vi "Day 07 (Part Two).vi"() -> ()   [LabVIEW 2021]
uses:
  4279ecf5-67f9-43a7-b6b3-78b14aefd003.vi
  4046d748-ad09-4f5d-82b9-a1e726cceff7.vi
  <userlib>/_OpenG.lib/array/array.llb/Sort 2D Array (I32)__ogtk.vi
  <vilib>/Comparison/Less/Less Functor/Less Functor.lvclass
panel:
  out "result":i32
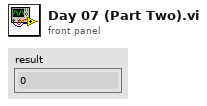
[diagram p1: front panel]
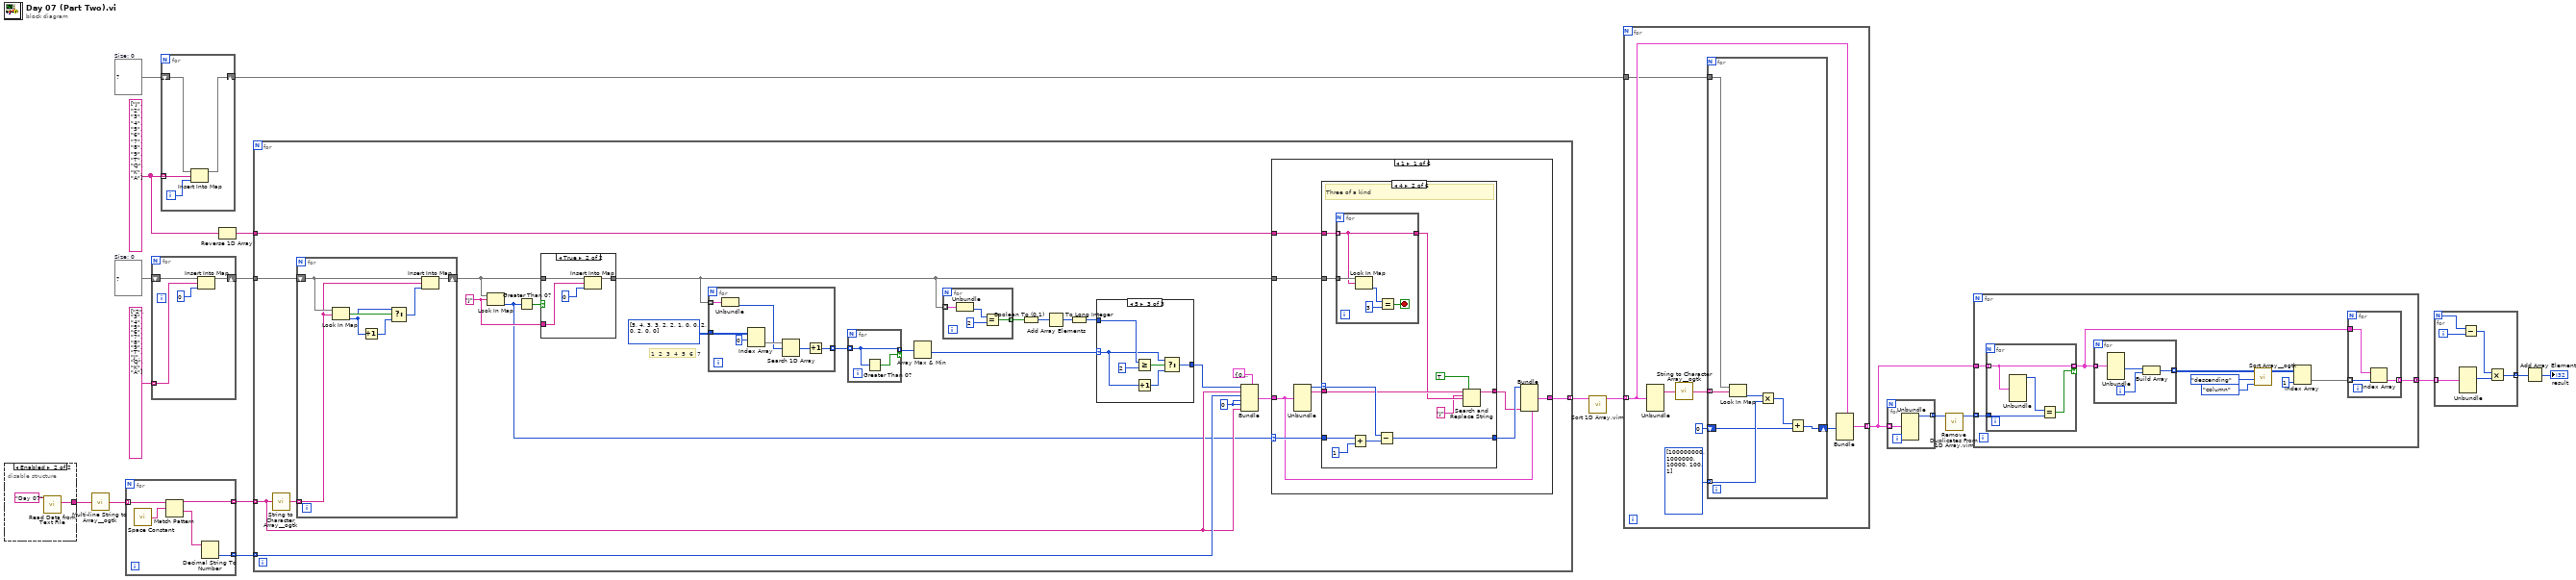
[diagram p0: block diagram]
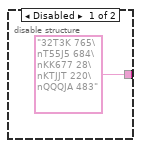
[diagram p2: hidden frame]
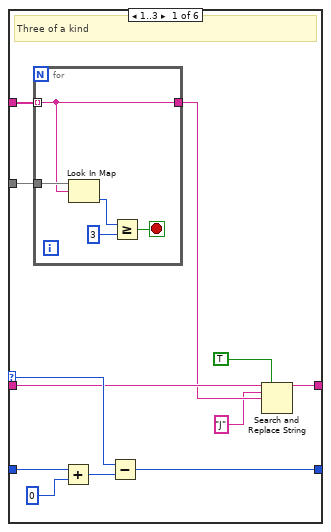
[diagram p3: hidden frame]
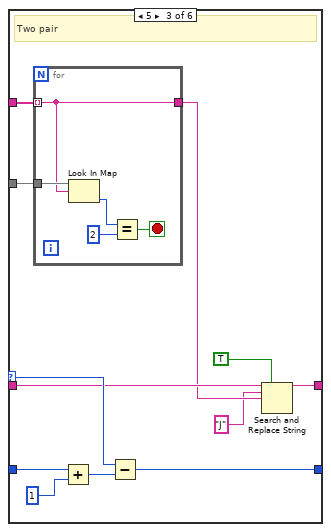
[diagram p4: hidden frame]
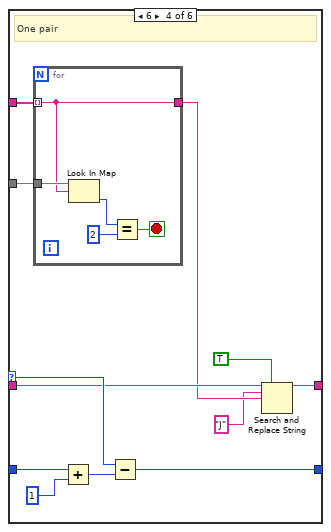
[diagram p5: hidden frame]
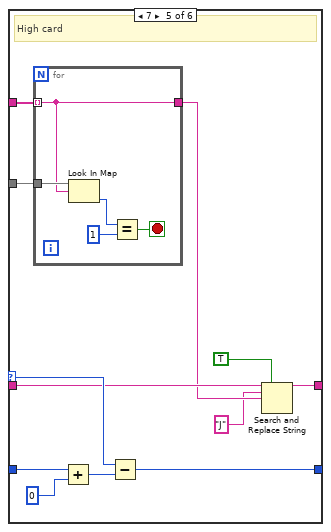
[diagram p6: hidden frame]
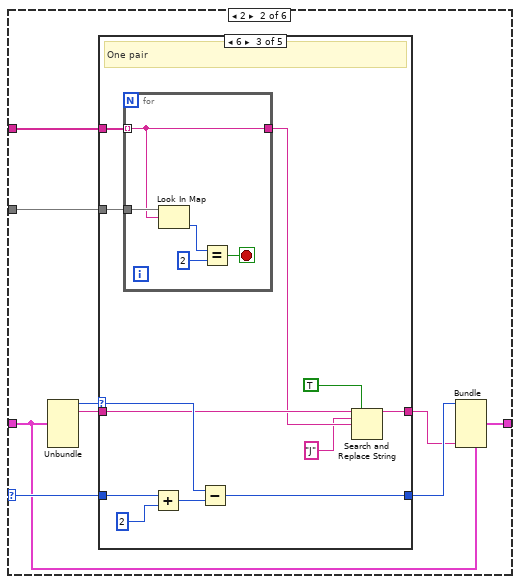
[diagram p8: hidden frame]
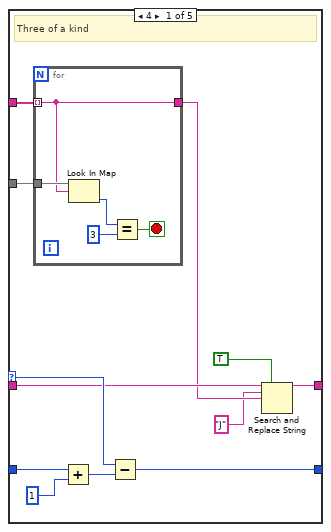
[diagram p9: hidden frame]
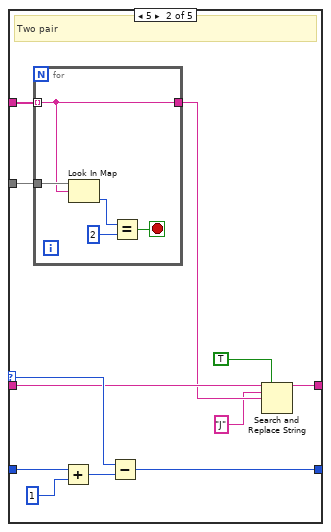
[diagram p10: hidden frame]
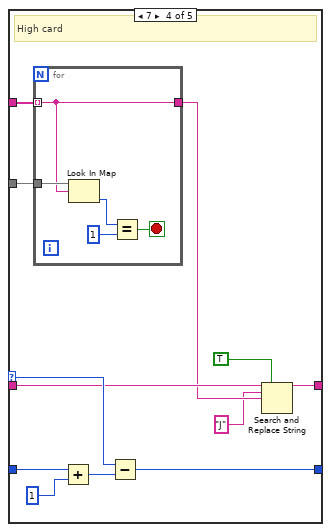
[diagram p11: hidden frame]
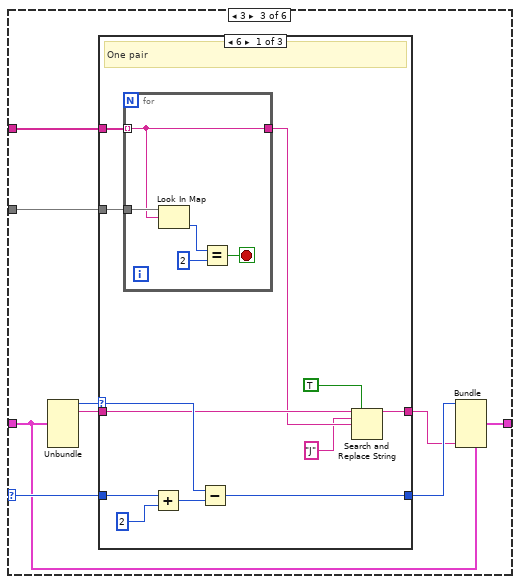
[diagram p13: hidden frame]
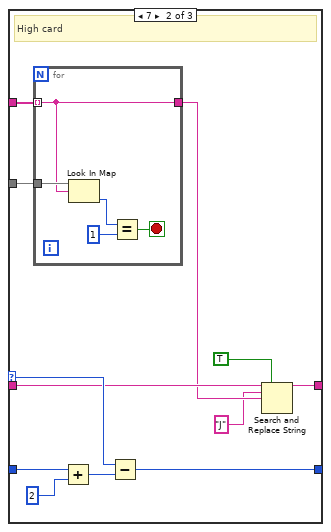
[diagram p14: hidden frame]
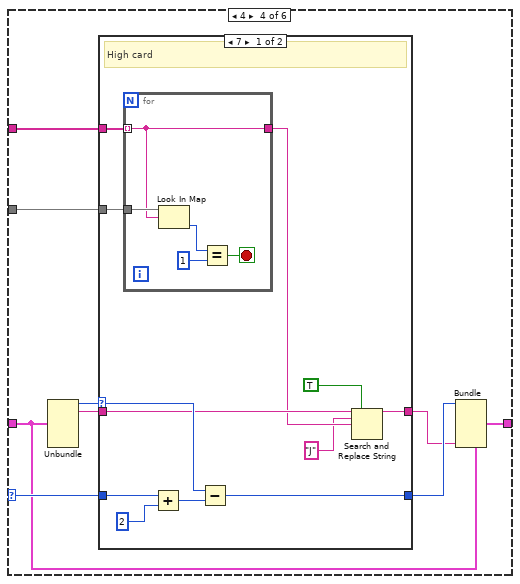
[diagram p16: hidden frame]
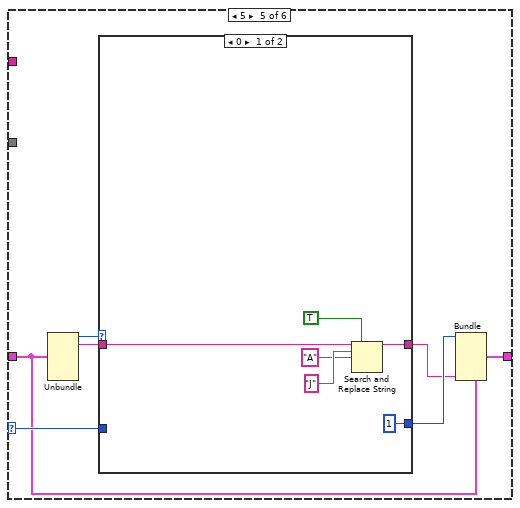
[diagram p18: hidden frame]
diagram:
  w2 = string[] ["J", "2", "3", "4", "5", "6", "7", "8", "9", "T", "Q", "K", "A"]
  w4 = map{string, i32} {}  # Size: 0
  w16 = map{string, i32} {}  # Size: 0
  n1 = disable-structure shown="Enabled" {
    disable-tunnel: ["32T3K 765\nT55J5 684\nKK677 28\nKTJJT 220\nQQQJA 483" w22] -> w19
    frame Disabled {
    }
    frame Enabled {
      n2 = call "Read Data from Text File.vi"("Subfolder"="Day 07") -> ("data"=w22:string)  [unwired: 10 in]
    }
  }
  n3 = call <userlib>:"Multi-line String to Array__ogtk.vi"("string"=w19) -> ("lines"=w18:string[])
  n4 = for {
    tunnel: w18 -> [w27] mode=indexing
    tunnel: [w25] -> w17 mode=indexing
    tunnel: [w23] -> w14 mode=indexing
    n5 = call <vilib>:"Space Constant.vi"() -> ("String"=w26:string)
    n6 = Match Pattern(string=w27, regular expression=w26) -> (before substring=w25:string, after substring=w24:string)  [unwired: 1 in, 2 out]
    n7 = Decimal String To Number(string=w24) -> (number=w23:i32)  [unwired: 2 in, 1 out]
  }
  n8 = for {
    shift-right: [w30] -> w5
    shift-left: w16 -> [w31]
    tunnel: string[] ["2", "3", "4", "5", "6", "7", "8", "9", "T", "J", "Q", "K", "A"] -> [w28] mode=indexing
    n9 = Insert Into Map(map in=w31, key=w28, value=0) -> (map out=w30:map{string, i32})  [unwired: 2 out]
  }
  n10 = for {
    shift-right: [w33] -> w3
    shift-left: w4 -> [w34]
    tunnel: w2 -> [w35] mode=indexing
    i -> [w32]
    n11 = Insert Into Map(map in=w34, key=w35, value=w32) -> (map out=w33:map{string, i32})  [unwired: 2 out]
  }
  n12 = Reverse 1D Array(array=w2) -> (reversed array=w1:string[])
  n13 = for {
    tunnel: w17 -> [w41] mode=indexing
    tunnel: w5 -> [w57]
    tunnel: [w38] -> w15 mode=indexing
    tunnel: w14 -> [w52] mode=indexing
    tunnel: w1 -> [w36]
    w45 = "J" ("key")
    w47 = 0
    # "1  2  3  4  5  6  7"
    n14 = call <userlib>:"String to Character Array__ogtk.vi"("Input String"=w41) -> ("Character Array"=w58:string[])
    n15 = for {
      tunnel: w58 -> [w315] mode=indexing
      shift-right: [w313] -> w44
      shift-left: w57 -> [w316]
      n16 = Look In Map(map=w316, key=w315) -> (key not found?=w319:bool, value=w317:i32)  [unwired: 1 in]
      n17 = Increment(x=w317) -> (x+1=w318:i32)
      n18 = Select(t=w317, s=w319, f=w318) -> (s? t:f=w314:i32)
      n19 = Insert Into Map(map in=w316, key=w315, value=w314) -> (map out=w313:map{string, i32})  [unwired: 2 out]
    }
    n20 = Look In Map(map=w44, key=w45) -> (value=w40:i32)  [unwired: 1 in, 1 out]
    n21 = Greater Than 0?(x=w40) -> (x > 0?=w46:bool)
    n22 = case shown="True" w46 {
      tunnel: w44 -> [w320 w324]
      tunnel: [w320 w323] -> w37
      tunnel: w45 -> [_ w322]
      frame False {
      }
      frame True {
        n23 = Insert Into Map(map in=w324, key=w322, value=0) -> (map out=w323:map{string, i32})  [unwired: 2 out]
      }
    }
    n24 = for {
      tunnel: w37 -> [w331] mode=indexing
      tunnel: i32[][] [[5, 4, 3, 3, 2, 2, 1], [0, 0, 2, 0, 2, 0, 0]] -> [w330]
      tunnel: [w325] -> w56 mode=indexing
      n25 = Unbundle(w331) -> (w327:i32)  [unwired: 1 out]
      n26 = Index Array(array=w330, index (row)=0) -> (element=w328:i32[])  [unwired: 1 in]
      n27 = Search 1D Array(1D array=w328, element=w327) -> (index of element=w326:i32)  [unwired: 1 in]
      n28 = Increment(x=w326) -> (x+1=w325:i32)
    }
    n29 = for {
      tunnel: w56 -> [w333] mode=indexing
      tunnel: [w333] -> w55 mode=indexing if=w332
      n30 = Greater Than 0?(x=w333) -> (x > 0?=w332:bool)
    }
    n31 = Array Max & Min(array=w55) -> (min value=w43:i32)  [unwired: 3 out]
    n32 = for {
      tunnel: w37 -> [w350] mode=indexing
      tunnel: [w347] -> w51 mode=indexing
      n33 = Unbundle(w350) -> (w349:i32)  [unwired: 1 out]
      n34 = Equal?(x=w349, y=2) -> (x = y?=w347:bool)
    }
    n35 = Boolean To (0,1)(Boolean=w51) -> (0, 1=w50:i16[])
    n36 = Add Array Elements(numeric array=w50) -> (sum=w49:i16)
    n37 = To Long Integer(number=w49) -> (32bit integer=w48:i32)
    n38 = case shown="5" w43 {
      selector: w43 -> [w334 w336 w342]
      tunnel: w48 -> [_ w339 w345]
      tunnel: [w334 w335 w341] -> w42
      frame Default {
      }
      frame 3 {
        n39 = Greater Or Equal?(x=w339, y=1) -> (x >= y?=w337:bool)
        n40 = Increment(x=w336) -> (x+1=w338:i32)
        n41 = Select(t=w336, s=w337, f=w338) -> (s? t:f=w335:i32)
      }
      frame 5 {
        n42 = Greater Or Equal?(x=w345, y=2) -> (x >= y?=w343:bool)
        n43 = Increment(x=w342) -> (x+1=w344:i32)
        n44 = Select(t=w342, s=w343, f=w344) -> (s? t:f=w341:i32)
      }
    }
    n45 = Bundle(cluster=cluster{i32, string, i32, i32, i32, string} {0, "", 0, 0, 0, ""}, w42, w41, w52, w47, w47, w41) -> (w39:cluster{i32, string, i32, i32, i32, string})
    n46 = case shown="1" w40 {
      selector: w40 -> [w66 w160 w237 w280 w304 _]
      tunnel: w39 -> [w63 w157 w234 w277 w302 w312]
      tunnel: [w60 w154 w231 w274 w299 w312] -> w38
      tunnel: w37 -> [w65 w159 w236 w279 _ _]
      tunnel: w36 -> [w59 w153 w230 w273 _ _]
      frame 1 {
        n47 = Unbundle(w63) -> (w67:i32, w64:string)  [unwired: 4 out]
        n48 = case shown="4" w67 {
          selector: w67 -> [w78 w95 w112 w129 w146 _]
          tunnel: w66 -> [w71 w88 w105 w122 w139 _]
          tunnel: w65 -> [w79 w96 w113 w130 w147 _]
          tunnel: w64 -> [w77 w94 w111 w128 w145 _]
          tunnel: [w73 w90 w107 w124 w141 _] -> w61
          tunnel: [w72 w89 w106 w123 w140 _] -> w62
          tunnel: w59 -> [w68 w85 w102 w119 w136 _]
          frame 1..3 {
            # "Three of a kind"
            n49 = for {
              tunnel: [w81] -> w76
              tunnel: w79 -> [w83]
              tunnel: w68 -> [w81] mode=indexing
              stop <- w80 stop-if-true
              n50 = Look In Map(map=w83, key=w81) -> (value=w82:i32)  [unwired: 1 in, 1 out]
              n51 = Greater Or Equal?(x=w82, y=3) -> (x >= y?=w80:bool)
            }
            n52 = Add(x=w71, y=0) -> (x+y=w70:i32)
            n53 = Subtract(x=w78, y=w70) -> (x-y=w72:i32)
            n54 = Search and Replace String(replace all?=TRUE ("replace all? (F)"), input string=w77, search string="J", replace string=w76) -> (result string=w73:string)  [unwired: 4 in, 3 out]
          }
          frame 4 {
            # "Three of a kind"
            n55 = for {
              tunnel: [w98] -> w93
              tunnel: w96 -> [w100]
              tunnel: w85 -> [w98] mode=indexing
              stop <- w97 stop-if-true
              n56 = Look In Map(map=w100, key=w98) -> (value=w99:i32)  [unwired: 1 in, 1 out]
              n57 = Equal?(x=w99, y=3) -> (x = y?=w97:bool)
            }
            n58 = Add(x=w88, y=1) -> (x+y=w87:i32)
            n59 = Subtract(x=w95, y=w87) -> (x-y=w89:i32)
            n60 = Search and Replace String(replace all?=TRUE ("replace all? (F)"), input string=w94, search string="J", replace string=w93) -> (result string=w90:string)  [unwired: 4 in, 3 out]
          }
          frame 5 {
            # "Two pair"
            n61 = for {
              tunnel: [w115] -> w110
              tunnel: w113 -> [w117]
              tunnel: w102 -> [w115] mode=indexing
              stop <- w114 stop-if-true
              n62 = Look In Map(map=w117, key=w115) -> (value=w116:i32)  [unwired: 1 in, 1 out]
              n63 = Equal?(x=w116, y=2) -> (x = y?=w114:bool)
            }
            n64 = Add(x=w105, y=1) -> (x+y=w104:i32)
            n65 = Subtract(x=w112, y=w104) -> (x-y=w106:i32)
            n66 = Search and Replace String(replace all?=TRUE ("replace all? (F)"), input string=w111, search string="J", replace string=w110) -> (result string=w107:string)  [unwired: 4 in, 3 out]
          }
          frame 6 {
            # "One pair"
            n67 = for {
              tunnel: [w132] -> w127
              tunnel: w130 -> [w134]
              tunnel: w119 -> [w132] mode=indexing
              stop <- w131 stop-if-true
              n68 = Look In Map(map=w134, key=w132) -> (value=w133:i32)  [unwired: 1 in, 1 out]
              n69 = Equal?(x=w133, y=2) -> (x = y?=w131:bool)
            }
            n70 = Add(x=w122, y=1) -> (x+y=w121:i32)
            n71 = Subtract(x=w129, y=w121) -> (x-y=w123:i32)
            n72 = Search and Replace String(replace all?=TRUE ("replace all? (F)"), input string=w128, search string="J", replace string=w127) -> (result string=w124:string)  [unwired: 4 in, 3 out]
          }
          frame 7 {
            # "High card"
            n73 = for {
              tunnel: [w149] -> w144
              tunnel: w147 -> [w151]
              tunnel: w136 -> [w149] mode=indexing
              stop <- w148 stop-if-true
              n74 = Look In Map(map=w151, key=w149) -> (value=w150:i32)  [unwired: 1 in, 1 out]
              n75 = Equal?(x=w150, y=1) -> (x = y?=w148:bool)
            }
            n76 = Add(x=w139, y=0) -> (x+y=w138:i32)
            n77 = Subtract(x=w146, y=w138) -> (x-y=w140:i32)
            n78 = Search and Replace String(replace all?=TRUE ("replace all? (F)"), input string=w145, search string="J", replace string=w144) -> (result string=w141:string)  [unwired: 4 in, 3 out]
          }
          frame Default {
          }
        }
        n79 = Bundle(cluster=w63, w62, w61) -> (w60:cluster{i32, string, i32, i32, i32, string})  [unwired: 4 in]
      }
      frame 2 {
        n80 = Unbundle(w157) -> (w161:i32, w158:string)  [unwired: 4 out]
        n81 = case shown="6" w161 {
          selector: w161 -> [w172 w189 w206 w223 _]
          tunnel: w160 -> [w165 w182 w199 w216 _]
          tunnel: w159 -> [w173 w190 w207 w224 _]
          tunnel: w158 -> [w171 w188 w205 w222 _]
          tunnel: [w167 w184 w201 w218 _] -> w155
          tunnel: [w166 w183 w200 w217 _] -> w156
          tunnel: w153 -> [w162 w179 w196 w213 _]
          frame 4 {
            # "Three of a kind"
            n82 = for {
              tunnel: [w175] -> w170
              tunnel: w173 -> [w177]
              tunnel: w162 -> [w175] mode=indexing
              stop <- w174 stop-if-true
              n83 = Look In Map(map=w177, key=w175) -> (value=w176:i32)  [unwired: 1 in, 1 out]
              n84 = Equal?(x=w176, y=3) -> (x = y?=w174:bool)
            }
            n85 = Add(x=w165, y=1) -> (x+y=w164:i32)
            n86 = Subtract(x=w172, y=w164) -> (x-y=w166:i32)
            n87 = Search and Replace String(replace all?=TRUE ("replace all? (F)"), input string=w171, search string="J", replace string=w170) -> (result string=w167:string)  [unwired: 4 in, 3 out]
          }
          frame 5 {
            # "Two pair"
            n88 = for {
              tunnel: [w192] -> w187
              tunnel: w190 -> [w194]
              tunnel: w179 -> [w192] mode=indexing
              stop <- w191 stop-if-true
              n89 = Look In Map(map=w194, key=w192) -> (value=w193:i32)  [unwired: 1 in, 1 out]
              n90 = Equal?(x=w193, y=2) -> (x = y?=w191:bool)
            }
            n91 = Add(x=w182, y=1) -> (x+y=w181:i32)
            n92 = Subtract(x=w189, y=w181) -> (x-y=w183:i32)
            n93 = Search and Replace String(replace all?=TRUE ("replace all? (F)"), input string=w188, search string="J", replace string=w187) -> (result string=w184:string)  [unwired: 4 in, 3 out]
          }
          frame 6 {
            # "One pair"
            n94 = for {
              tunnel: [w209] -> w204
              tunnel: w207 -> [w211]
              tunnel: w196 -> [w209] mode=indexing
              stop <- w208 stop-if-true
              n95 = Look In Map(map=w211, key=w209) -> (value=w210:i32)  [unwired: 1 in, 1 out]
              n96 = Equal?(x=w210, y=2) -> (x = y?=w208:bool)
            }
            n97 = Add(x=w199, y=2) -> (x+y=w198:i32)
            n98 = Subtract(x=w206, y=w198) -> (x-y=w200:i32)
            n99 = Search and Replace String(replace all?=TRUE ("replace all? (F)"), input string=w205, search string="J", replace string=w204) -> (result string=w201:string)  [unwired: 4 in, 3 out]
          }
          frame 7 {
            # "High card"
            n100 = for {
              tunnel: [w226] -> w221
              tunnel: w224 -> [w228]
              tunnel: w213 -> [w226] mode=indexing
              stop <- w225 stop-if-true
              n101 = Look In Map(map=w228, key=w226) -> (value=w227:i32)  [unwired: 1 in, 1 out]
              n102 = Equal?(x=w227, y=1) -> (x = y?=w225:bool)
            }
            n103 = Add(x=w216, y=1) -> (x+y=w215:i32)
            n104 = Subtract(x=w223, y=w215) -> (x-y=w217:i32)
            n105 = Search and Replace String(replace all?=TRUE ("replace all? (F)"), input string=w222, search string="J", replace string=w221) -> (result string=w218:string)  [unwired: 4 in, 3 out]
          }
          frame Default {
          }
        }
        n106 = Bundle(cluster=w157, w156, w155) -> (w154:cluster{i32, string, i32, i32, i32, string})  [unwired: 4 in]
      }
      frame 3 {
        n107 = Unbundle(w234) -> (w238:i32, w235:string)  [unwired: 4 out]
        n108 = case shown="6" w238 {
          selector: w238 -> [w249 w266 _]
          tunnel: w237 -> [w242 w259 _]
          tunnel: w236 -> [w250 w267 _]
          tunnel: w235 -> [w248 w265 _]
          tunnel: [w244 w261 _] -> w232
          tunnel: [w243 w260 _] -> w233
          tunnel: w230 -> [w239 w256 _]
          frame 6 {
            # "One pair"
            n109 = for {
              tunnel: [w252] -> w247
              tunnel: w250 -> [w254]
              tunnel: w239 -> [w252] mode=indexing
              stop <- w251 stop-if-true
              n110 = Look In Map(map=w254, key=w252) -> (value=w253:i32)  [unwired: 1 in, 1 out]
              n111 = Equal?(x=w253, y=2) -> (x = y?=w251:bool)
            }
            n112 = Add(x=w242, y=2) -> (x+y=w241:i32)
            n113 = Subtract(x=w249, y=w241) -> (x-y=w243:i32)
            n114 = Search and Replace String(replace all?=TRUE ("replace all? (F)"), input string=w248, search string="J", replace string=w247) -> (result string=w244:string)  [unwired: 4 in, 3 out]
          }
          frame 7 {
            # "High card"
            n115 = for {
              tunnel: [w269] -> w264
              tunnel: w267 -> [w271]
              tunnel: w256 -> [w269] mode=indexing
              stop <- w268 stop-if-true
              n116 = Look In Map(map=w271, key=w269) -> (value=w270:i32)  [unwired: 1 in, 1 out]
              n117 = Equal?(x=w270, y=1) -> (x = y?=w268:bool)
            }
            n118 = Add(x=w259, y=2) -> (x+y=w258:i32)
            n119 = Subtract(x=w266, y=w258) -> (x-y=w260:i32)
            n120 = Search and Replace String(replace all?=TRUE ("replace all? (F)"), input string=w265, search string="J", replace string=w264) -> (result string=w261:string)  [unwired: 4 in, 3 out]
          }
          frame Default {
          }
        }
        n121 = Bundle(cluster=w234, w233, w232) -> (w231:cluster{i32, string, i32, i32, i32, string})  [unwired: 4 in]
      }
      frame 4 {
        n122 = Unbundle(w277) -> (w281:i32, w278:string)  [unwired: 4 out]
        n123 = case shown="7" w281 {
          selector: w281 -> [w292 _]
          tunnel: w280 -> [w285 _]
          tunnel: w279 -> [w293 _]
          tunnel: w278 -> [w291 _]
          tunnel: [w287 _] -> w275
          tunnel: [w286 _] -> w276
          tunnel: w273 -> [w282 _]
          frame 7 {
            # "High card"
            n124 = for {
              tunnel: [w295] -> w290
              tunnel: w293 -> [w297]
              tunnel: w282 -> [w295] mode=indexing
              stop <- w294 stop-if-true
              n125 = Look In Map(map=w297, key=w295) -> (value=w296:i32)  [unwired: 1 in, 1 out]
              n126 = Equal?(x=w296, y=1) -> (x = y?=w294:bool)
            }
            n127 = Add(x=w285, y=2) -> (x+y=w284:i32)
            n128 = Subtract(x=w292, y=w284) -> (x-y=w286:i32)
            n129 = Search and Replace String(replace all?=TRUE ("replace all? (F)"), input string=w291, search string="J", replace string=w290) -> (result string=w287:string)  [unwired: 4 in, 3 out]
          }
          frame Default {
          }
        }
        n130 = Bundle(cluster=w277, w276, w275) -> (w274:cluster{i32, string, i32, i32, i32, string})  [unwired: 4 in]
      }
      frame 5 {
        n131 = Unbundle(w302) -> (w305:i32, w303:string)  [unwired: 4 out]
        n132 = case shown="0" w305 {
          tunnel: w304 -> [_ _]
          tunnel: w303 -> [w311 _]
          tunnel: [w308 _] -> w300
          tunnel: [1 _] -> w301
          frame 0 {
            n133 = Search and Replace String(replace all?=TRUE ("replace all? (F)"), input string=w311, search string="J", replace string="A" ("search string")) -> (result string=w308:string)  [unwired: 4 in, 3 out]
          }
          frame Default {
          }
        }
        n134 = Bundle(cluster=w302, w301, w300) -> (w299:cluster{i32, string, i32, i32, i32, string})  [unwired: 4 in]
      }
      frame Default {
      }
    }
  }
  n135 = call "Sort 1D Array.vim"("unsorted array"=w15) -> ("sorted array"=w13:cluster{i32, string, i32, i32, i32, string}[])  [unwired: 10 in]
  n136 = for {
    tunnel: w13 -> [w355] mode=indexing
    tunnel: [w353] -> w10 mode=indexing
    tunnel: w3 -> [w352]
    n137 = Unbundle(w355) -> (w351:string)  [unwired: 5 out]
    n138 = call <userlib>:"String to Character Array__ogtk.vi"("Input String"=w351) -> ("Character Array"=w358:string[])
    n139 = for {
      tunnel: w358 -> [w363] mode=indexing
      tunnel: i32[] [100000000, 1000000, 10000, 100, 1] -> [w364] mode=indexing
      shift-right: [w362] -> w354
      shift-left: 0 -> [w360]
      tunnel: w352 -> [w359]
      n140 = Look In Map(map=w359, key=w363) -> (value=w365:i32)  [unwired: 1 in, 1 out]
      n141 = Multiply(x=w365, y=w364) -> (x*y=w361:i32)
      n142 = Add(x=w361, y=w360) -> (x+y=w362:i32)
    }
    n143 = Bundle(cluster=w355, w354) -> (w353:cluster{i32, string, i32, i32, i32, string})  [unwired: 5 in]
  }
  n144 = for {
    tunnel: w10 -> [w367] mode=indexing
    tunnel: [w366] -> w12 mode=indexing
    n145 = Unbundle(w367) -> (w366:i32)  [unwired: 5 out]
  }
  n146 = call "Remove Duplicates From 1D Array.vim"("array"=w12) -> ("array with duplicates removed"=w11:i32[])  [unwired: 10 in]
  n147 = for {
    tunnel: w11 -> [w376] mode=indexing
    tunnel: w10 -> [w377]
    tunnel: [w368] -> w9 mode=concatenating
    n148 = for {
      tunnel: w377 -> [w379] mode=indexing
      tunnel: w376 -> [w380]
      tunnel: [w379] -> w369 mode=indexing if=w378
      n149 = Unbundle(w379) -> (w381:i32)  [unwired: 5 out]
      n150 = Equal?(x=w381, y=w380) -> (x = y?=w378:bool)
    }
    n151 = for {
      tunnel: w369 -> [w388] mode=indexing
      tunnel: [w385] -> w375 mode=indexing
      i -> [w386]
      n152 = Unbundle(w388) -> (w387:i32)  [unwired: 5 out]
      n153 = Build Array(w387, w386) -> (w385:i32[])
    }
    n154 = call-poly <userlib>:"Sort Array__ogtk.vi"("Sort By in"=enum16{"row", "column"}."column", "Order"=enum16{"ascending", "descending"}."descending", "Array in"=w375) -> ("Sorted Array out"=w372:i32[][])  [unwired: 5 in, 3 out]
    n155 = Index Array(array=w372, index (col)=1 ("disabled index (col)")) -> (element=w370:i32[])  [unwired: 1 in]
    n156 = for {
      tunnel: w370 -> [w383] mode=indexing
      tunnel: w369 -> [w384]
      tunnel: [w382] -> w368 mode=indexing
      n157 = Index Array(array=w384, index=w383) -> (element=w382:cluster{i32, string, i32, i32, i32, string})
    }
  }
  n158 = for {
    N -> [w394]
    tunnel: w9 -> [w390] mode=indexing
    tunnel: [w389] -> w8 mode=indexing
    i -> [w393]
    n159 = Unbundle(w390) -> (w391:i32)  [unwired: 5 out]
    n160 = Subtract(x=w394, y=w393) -> (x-y=w392:i32)
    n161 = Multiply(x=w392, y=w391) -> (x*y=w389:i32)
  }
  n162 = Add Array Elements(numeric array=w8) -> (sum=→"result":i32)
